vi "Encode Compressed Message.vi"(8 "Compression (zip)":T1=enum."7z", 9 "Messages to Encode (-1)":i32=-1, 10 "Array To Encode":u8[](array[numeric]), 11 "Image In":u8[](array[numeric])) -> (2 "Bytes Free":i32, 3 "Image Out":u8[](array[numeric]))   [LabVIEW 2020]
uses:
  Compression Type.ctl
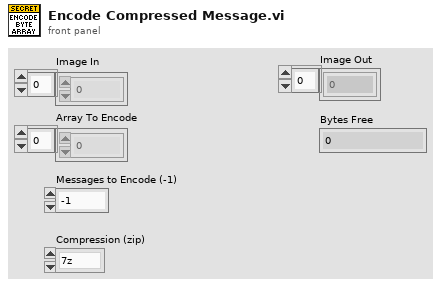
[diagram p1: front panel]
types:
  T1 = typedef "Compression Type.ctl" = enum8{"zip", "7z", "zpaq"}
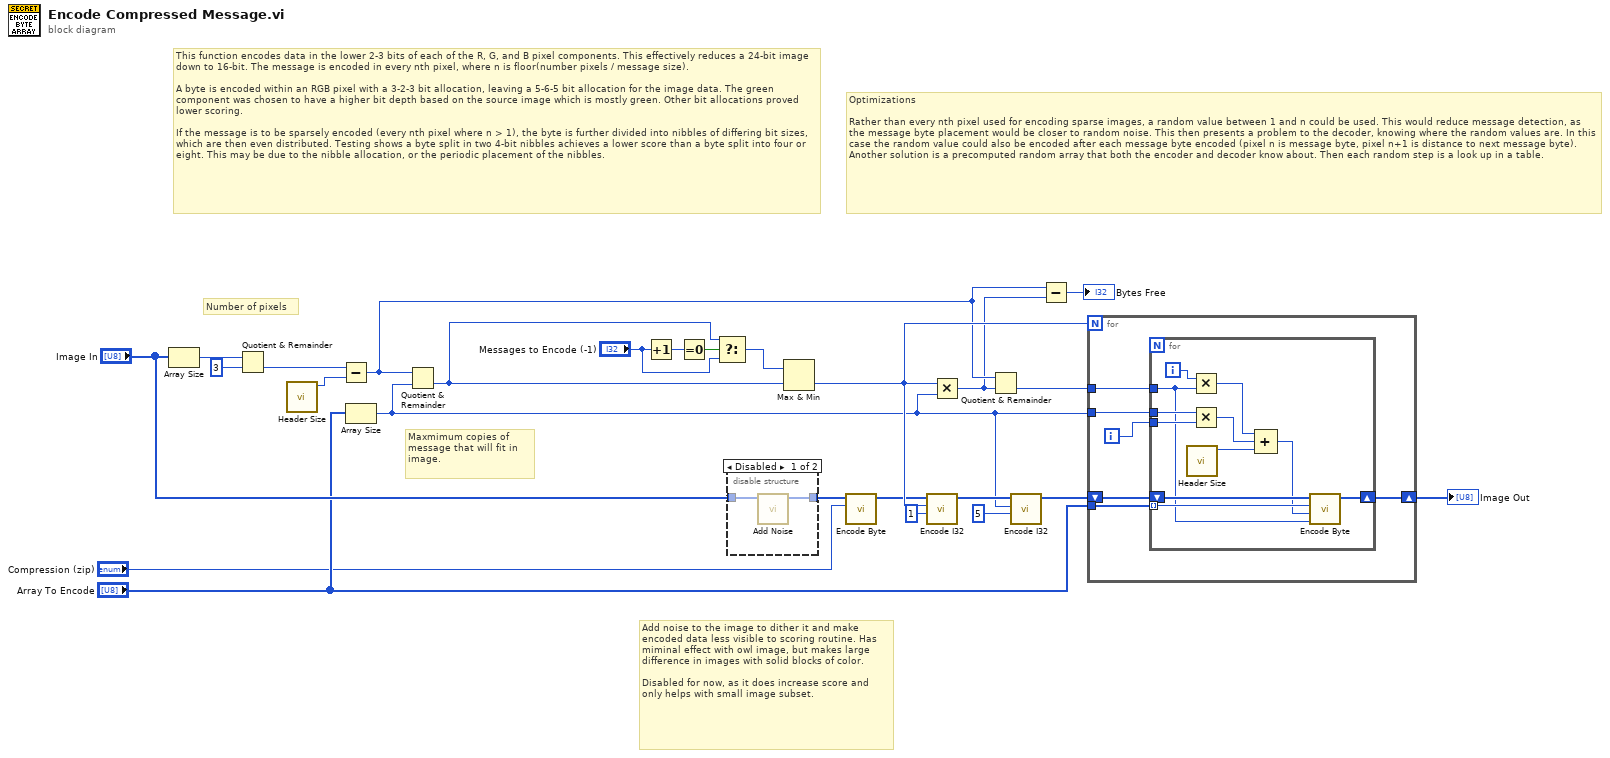
[diagram p0: block diagram]
diagram:
  # "Optimizations\n\nRather than every nth pixel used for encoding sparse images, a random value between 1 and n could be used. This would reduce message detection, as the message byte placement would be closer to random noise. This then presents a problem to the decoder, knowing where the random values are. In this case the random value could also be encoded after each message byte encoded (pixel n is message byte, pixel n+1 is distance to next message byte). Another solution is a precomputed random array that both the encoder and decoder know about. Then each random step is a look up in a table."
  # "This function encodes data in the lower 2-3 bits of each of the R, G, and B pixel components. This effectively reduces a 24-bit image down to 16-bit. The message is encoded in every nth pixel, where n is floor(number pixels / message size).\n\nA byte is encoded within an RGB pixel with a 3-2-3 bit allocation, leaving a 5-6-5 bit allocation for the image data. The green component was chosen to have a higher bit depth based on the source image which is mostly green. Other bit allocations proved lower scoring.\n\nIf the message is to be sparsely encoded (every nth pixel where n > 1), the byte is further divided into nibbles of differing bit sizes, which are then even distributed. Testing shows a byte split in two 4-bit nibbles achieves a lower score than a byte split into four or eight. This may be due to the nibble allocation, or the periodic placement of the nibbles."
  # "Add noise to the image to dither it and make encoded data less visible to scoring routine. Has miminal effect with owl image, but makes large difference in images with solid blocks of color.\n\nDisabled for now, as it does increase score and only helps with small image subset."
  # "Maxmimum copies of message that will fit in image."
  # "Number of pixels"
  n1 = Array Size(array="Image In") -> (size(s)=w25:i32)
  n2 = Quotient & Remainder(x=w25, y=3) -> (floor(x/y)=w22:i32)  [unwired: 1 out]
  n3 = call "Header Size.vi"() -> ("Header Size"=w1:i32)  [unwired: 11 in]
  n4 = Subtract(x=w22, y=w1) -> (x-y=w8:i32)
  n5 = Array Size(array="Array To Encode") -> (size(s)=w11:i32)
  n6 = Quotient & Remainder(x=w8, y=w11) -> (floor(x/y)=w18:i32)  [unwired: 1 out]
  n7 = Increment(x="Messages to Encode (-1)") -> (x+1=w21:i32)
  n8 = Equal To 0?(x=w21) -> (x = 0?=w20:bool)
  n9 = Select(t=w18, s=w20, f="Messages to Encode (-1)") -> (s? t:f=w15:i32)
  n10 = disable-structure shown="Disabled" {
    disable-tunnel: "Image In" -> [w27 w28]
    disable-tunnel: [w26 w28] -> w5
    frame Disabled {
      n11 = call "Add Noise.vi"("Image In"=w27) -> ("Image Out"=w26:u8[])  [unwired: 10 in]
    }
    frame Enabled {
    }
  }
  n12 = Max & Min(x=w15, y=w18) -> (min(x,y)=w13:i32)  [unwired: 1 out]
  n13 = call "Encode Byte.vi"("Byte To Encode"="Compression (zip)", "Image In"=w5) -> ("Image Out"=w4:u8[])  [unwired: 9 in]
  n14 = call "Encode I32.vi"("Pixel Offset (0)"=1, "I32"=w13, "Image In"=w4) -> ("Image Out"=w12:u8[])  [unwired: 8 in]
  n15 = Multiply(x=w13, y=w11) -> (x*y=w7:i32)
  n16 = Quotient & Remainder(x=w8, y=w7) -> (floor(x/y)=w16:i32)  [unwired: 1 out]
  n17 = call "Encode I32.vi"("Pixel Offset (0)"=5 ("y"), "I32"=w11, "Image In"=w12) -> ("Image Out"=w9:u8[])  [unwired: 8 in]
  n18 = Subtract(x=w8, y=w7) -> (x-y=→"Bytes Free":i32)
  n19 = for {
    N: w13 -> [_]
    tunnel: "Array To Encode" -> [w34]
    shift-right: [w33] -> w23
    shift-left: w9 -> [w32]
    tunnel: w11 -> [w30]
    tunnel: w16 -> [w29]
    i -> [w31]
    n20 = for {
      tunnel: w34 -> [w44] mode=indexing
      shift-right: [w42] -> w33
      shift-left: w32 -> [w45]
      tunnel: w31 -> [w41]
      tunnel: w30 -> [w40]
      tunnel: w29 -> [w35]
      i -> [w39]
      n21 = call "Header Size.vi"() -> ("Header Size"=w36:i32)  [unwired: 11 in]
      n22 = Multiply(x=w39, y=w35) -> (x*y=w38:i32)
      n23 = Multiply(x=w40, y=w41) -> (x*y=w37:i32)
      n24 = Compound Arithmetic op=ADD(w38, w37, w36) -> (w43:i32)
      n25 = call "Encode Byte.vi"("Step Size (1)"=w35, "Pixel Offset (0)"=w43, "Byte To Encode"=w44, "Image In"=w45) -> ("Image Out"=w42:u8[])  [unwired: 7 in]
    }
  }
  "Image Out" <- w23
